vi "to string.vi"(8 "error in":errorcluster, 11 "module configuration in":refnum<class "TBM module configuration.lvclass">) -> (0 "error out":errorcluster, 1 "data":string, 2 "version":string, 3 "module configuration out":refnum<class "TBM module configuration.lvclass">)   [LabVIEW 2013, in "TBM module configuration.lvclass"]
doc: "Provides an interface for saving a module configuration to a file or other serialized data source. It is recommended that all children of this class store data in two sets--data required for its own initialization, and any data required for parent initialization--and that each implementation uses the <b>Call Parent Method</b> primitive to serialize parent information."
uses:
  TBM module configuration.lvclass
  root configuration/TBM configuration.lvclass
  <vilib>/NI/CEF/CEF_TreeControl/serializable configuration/NISE_CEF_serializable configuration.lvclass
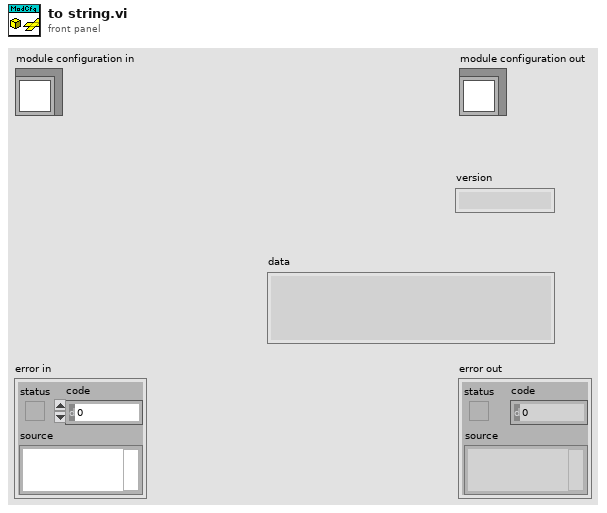
[diagram p1: front panel]
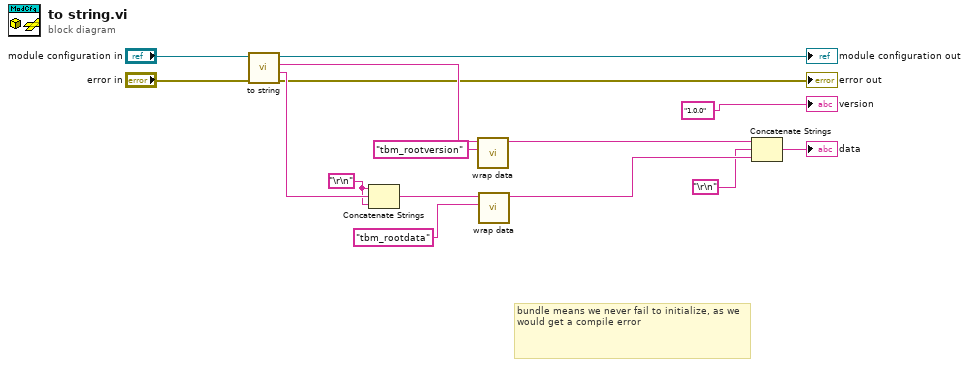
[diagram p0: block diagram]
diagram:
  w2 = "\r\n"
  # "bundle means we never fail to initialize, as we would get a compile error"
  n1 = call-parent "to string.vi"("error in"="error in", "configuration in"="module configuration in") -> ("error out"=→"error out":errorcluster, "data"=w9:string, "version"=w13:string, "configuration out"=→"module configuration out":refnum<class "TBM module configuration.lvclass">)  [unwired: 6 in]
  n2 = Concatenate Strings(w2, w9, w2) -> (w3:string)
  n3 = call <vilib>:"wrap data.vi"("identifier"="tbm_rootversion" ("additional identifier"), "data to wrap"=w13) -> ("wrapped data"=w7:string)  [unwired: 9 in]
  n4 = call <vilib>:"wrap data.vi"("identifier"="tbm_rootdata" ("additional identifier"), "data to wrap"=w3) -> ("wrapped data"=w8:string)  [unwired: 9 in]
  n5 = Concatenate Strings(w7, "\r\n", w8) -> (→"data":string)
  "version" <- "1.0.0" ("version 2")
